vi "Rectangular Target - 2013Vr2.vi"(3 "Camera Settings":T4={"FPS"=30, "Compression"=30, "Image Size"=enum."320x240"}, 4 "Target Choice":i8(knob) scale=0.0..2.0, 5 "Camera IP Address":string="192.168.0.90", 6 "Camera Image":T2(plugin-control)) -> (0 "Center Target":bool, 1 "Processed Image":T2(plugin-control), 2 "Numeric Target Info":dbl[](array[numeric]))   [LabVIEW 2012]
doc: "This VI demonstrates how to do target processing on a laptop computer. It uses the same MJPG VI as the dashboard, sets a few of the important camera properties that impact processing, and carries out the same processing steps as the RT example also included in this project."
uses:
  <vilib>/Rock Robotics/WPI/Camera/WPI_CameraImageSize.ctl
  <vilib>/Rock Robotics/WPI/Camera/WPI_CameraWhite Balance Values.ctl
  <vilib>/vision/NI_Vision_Development_Module.lvlib
panel:
  in  "Camera Settings 2":T1={"Frate Rate"=30, "Compression"=30, "Size"=1} {"Size" items=["640x480", "320x240", "160x120"]; "Frate Rate" scale=1.0..30.0}
  out "fps":dbl format="%#.1g"
  in  "Camera Type":enum16{"206", "1011"}(ring)=enum."1011"
  in  "Image Source":enum32{"Live Camera", "File Images"}(tab)
  in  "Directory":path
  in  "File List":i32(listbox)
  out "Target Info":T5(array[cluster])
  in  "Area Size Limit %":dbl=0.5
  in  "Particle Count Limit":i32=10
  in  "Score Limits":T6={"Rect Coverage"=60.0, "X Edge Strength"=40.0, "Y Edge Strength"=60.0, "Center"=75.0, "Outer"=75.0}
  in  "Processing":enum32{"Color", "Monochrome"}(tab)
  out "Value":cluster{i32, i32}
  out "Saturation":cluster{i32, i32}
  in  "Value":i32=255
  in  "Saturation":i32=255
  in  "Hue":i32(knob)=65 scale=0.0..255.0
  in  "Margins":cluster{"Hue":i32, "Sat":i32, "Val":i32}={"Hue"=33, "Sat"=53, "Val"=9} {"Sat" scale=0.0..80.0; "Val" scale=0.0..80.0; "Hue" scale=0.0..80.0}
  out "Hue":cluster{i32, i32}
  in  "Range":cluster{"Lower value":sgl, "Upper value":sgl}={"Lower value"=150.0, "Upper value"=255.0} {"Lower value" scale=0.0..255.0; "Upper value" scale=0.0..255.0}
  in  "Color Plane":i32(ring)=6 items=["Red", "Green", "Blue", "Hue", "Saturation", "Luminance", "Value", "Intensity"]
  in  "Annotate":bool=TRUE
  out "Original Image":T2(plugin-control)
  # "Information:\nProcessing can be based on color or light intensity.\nParticles within the image are scored by rectangle coverage, aspect ratio, and\nedge strength/hollowness. A particle is considered a target if all scores\nare above the score limits you set. Particles can be annotated -- surrounded by\na rectangle and scores drawn to the left .\nTo control the number of particles being scored, use the count limit and the size\nlimit.\nBe sure to set the Camera IP before running. The distance calculation uses the\ncamera type to index the value of the lens view angle."
  # "Click in the image to choose  color for processing."
  # "Green scores are above the limit, orange are below. Inner/outer rect\nindicates all passed."
  # "Set before running."
  # "Lower/Upper"
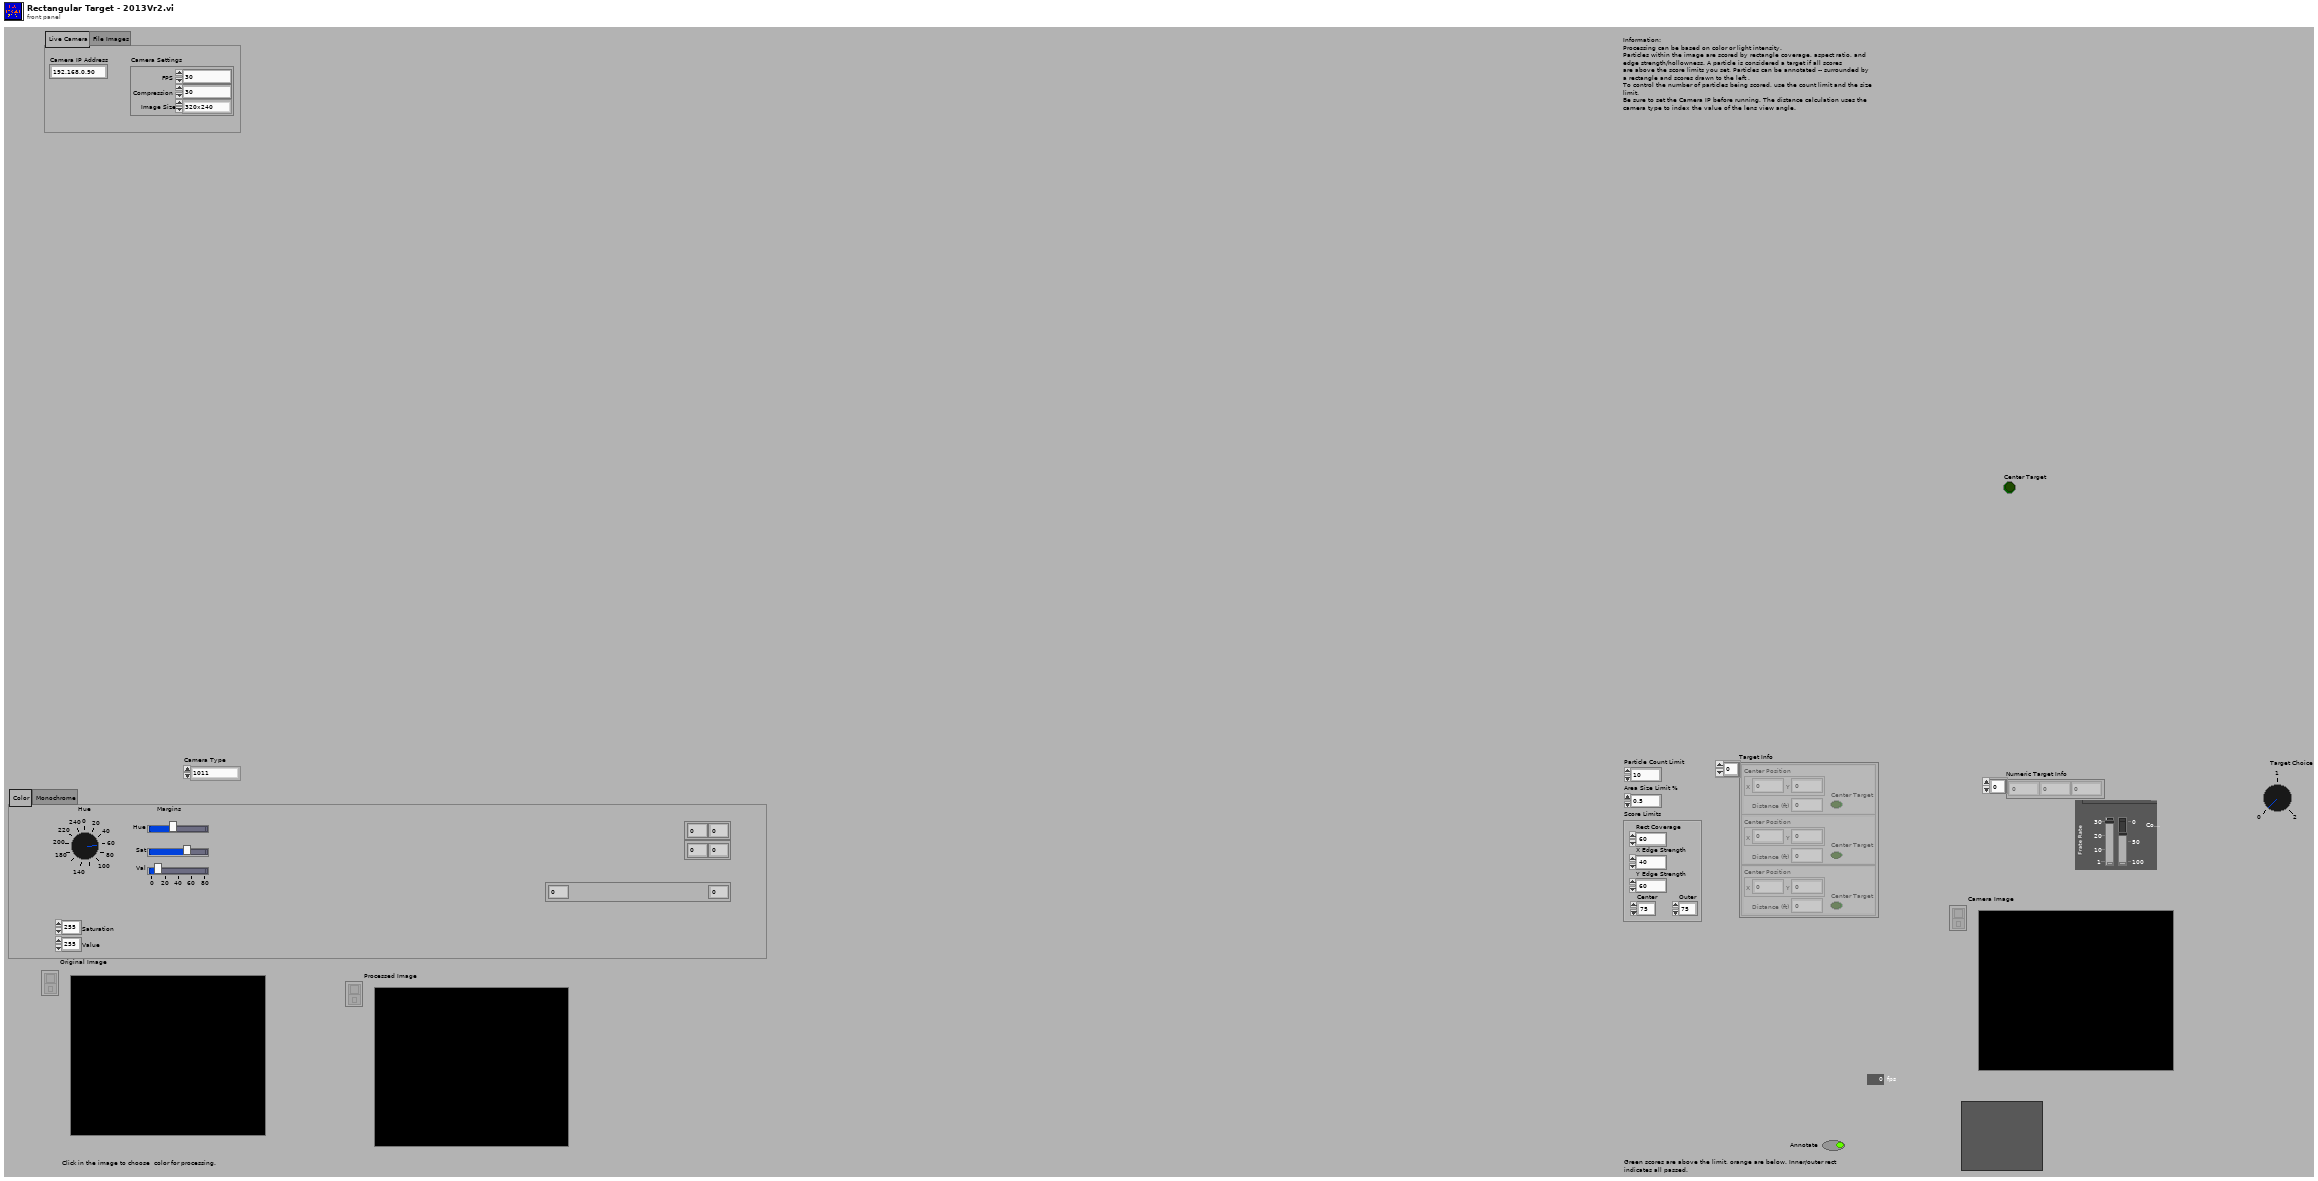
[diagram p1: front panel]
types:
  T1 = cluster{"Frate Rate":i32, "Compression":i32, "Size":u16}
  T2 = typedef "IMAQ Image.ctl" = refnum<image>
  T3 = typedef "WPI_CameraImageSize.ctl" = enum16{"640x480", "320x240", "160x120"}
  T4 = cluster{"FPS":i32, "Compression":i32, "Image Size":T3}
  T5 = cluster{"Center Position":cluster{"X":dbl, "Y":dbl}, "Distance (ft)":dbl, "Center Target":bool}[]
  T6 = cluster{"Rect Coverage":dbl, "X Edge Strength":dbl, "Y Edge Strength":dbl, "Center":dbl, "Outer":dbl}
  T7 = typedef "Image Type" = u32
  T8 = typedef "WPI_CameraWhite Balance Values.ctl" = enum16{"Auto", "Fixed indoor", "Fixed outdoor 1", "Fixed outdoor 2", "Fixed fluorescent 1", "Fixed fluorescent 2", "Hold current"}
  T9 = typedef "WPI_CameraDevRef.ctl" = cluster{"Camera Address":string, "CameraStatus":errorcluster, "Acquire Image Notifier":refnum<notifier>}
  T10 = cluster{"Position":cluster{"X":dbl, "Y":dbl}, "Distance (ft)":dbl, "Center Target":bool}[]
  T11 = cluster{cluster{"Left":dbl, "Top":dbl, "Right":dbl, "Bottom":dbl}, "Scores":dbl[], cluster{"Long":dbl, "Short":dbl}}[]
  T12 = cluster{"Target Center (-1 to 1)":cluster{"X":dbl, "Y":dbl}, "Distance (ft)":dbl, "Center Target":bool}
  T13 = cluster{"Target Center (-1 to 1)":cluster{"X":dbl, "Y":dbl}, "Distance (ft)":dbl, "Center Target":bool}[]
  T14 = cluster{"Left":dbl, "Top":dbl, "Right":dbl, "Bottom":dbl}
  T15 = cluster{"Position":cluster{"X":dbl, "Y":dbl}, "Distance (ft)":dbl, "Center Target":bool}
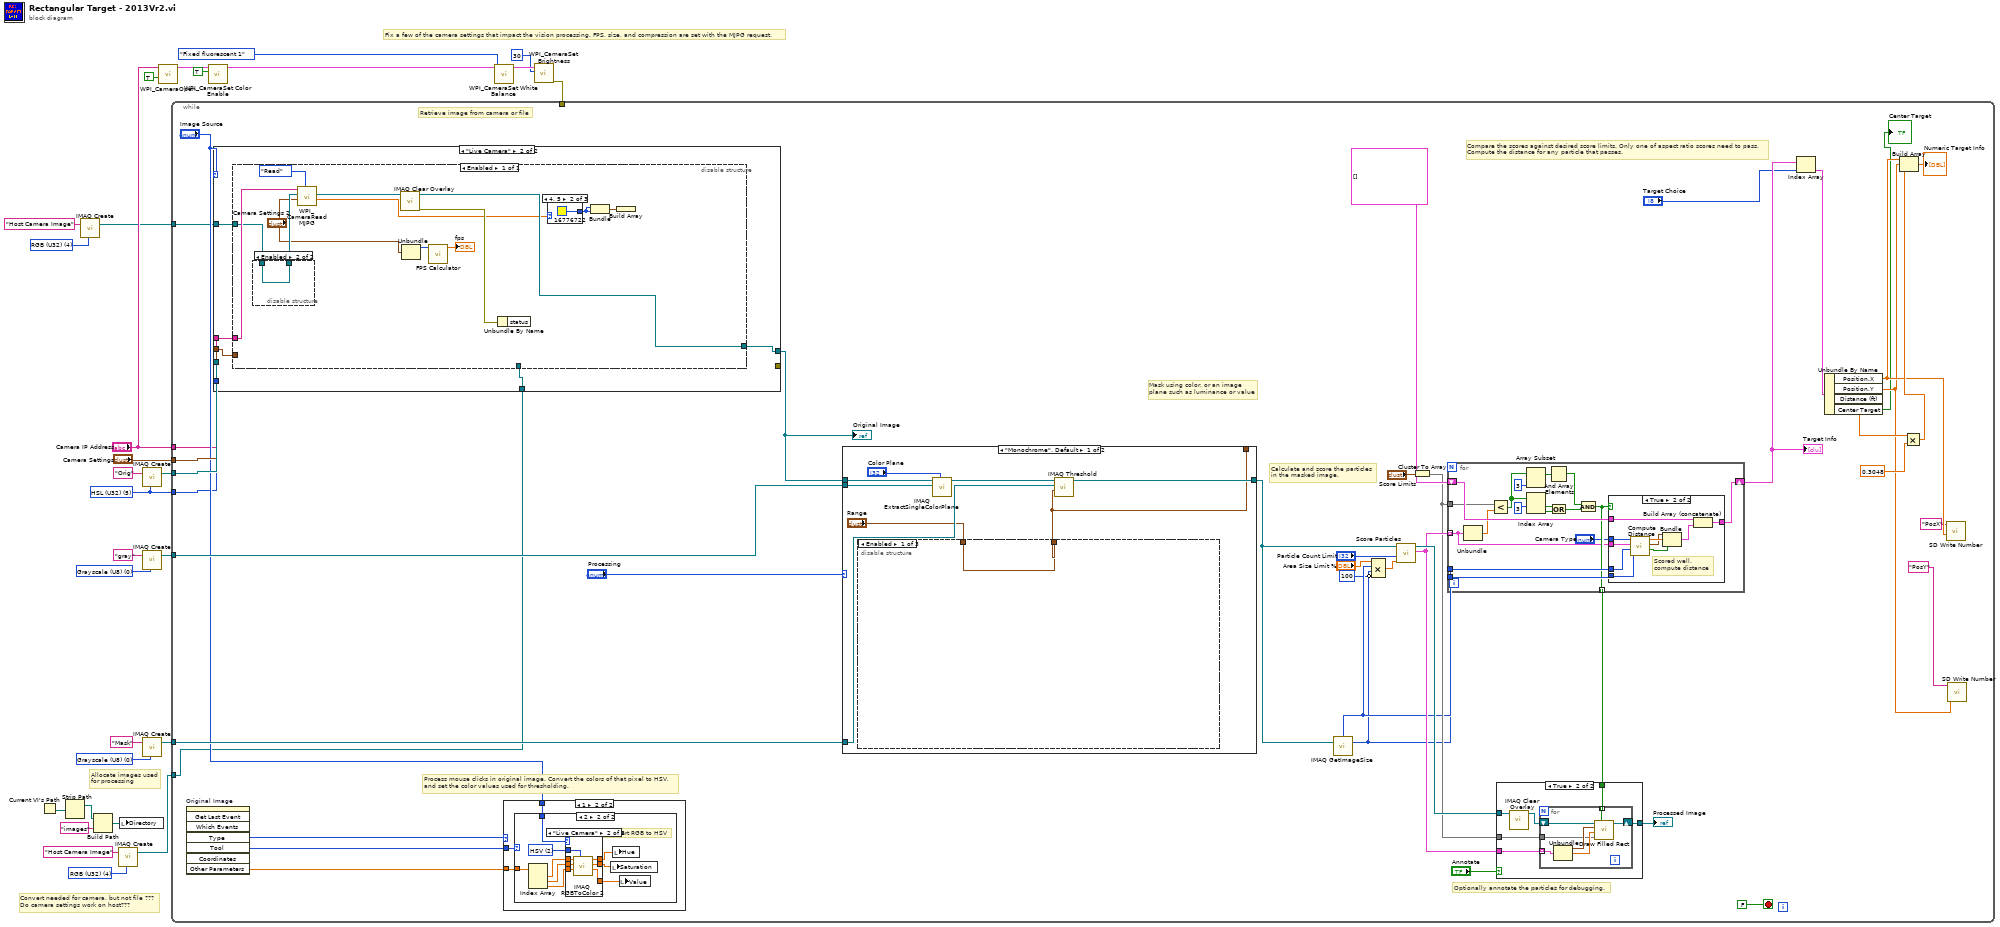
[diagram p0: block diagram]
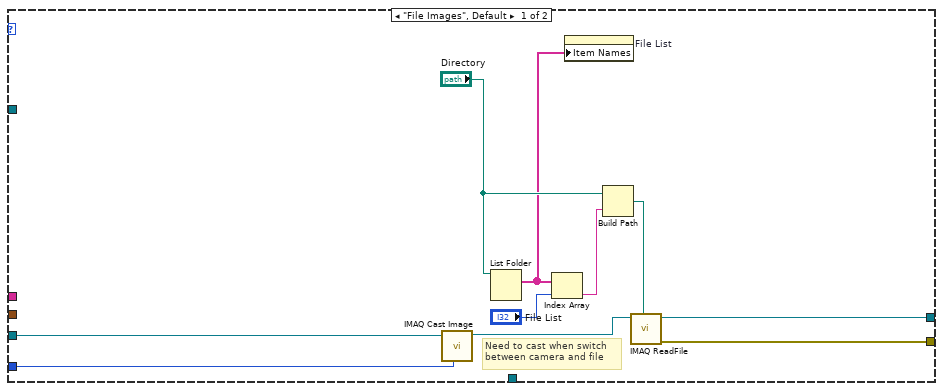
[diagram p2: hidden frame]
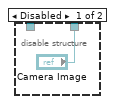
[diagram p3: hidden frame]
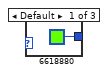
[diagram p4: hidden frame]
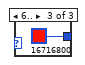
[diagram p5: hidden frame]
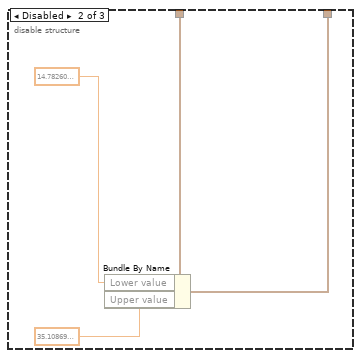
[diagram p7: hidden frame]
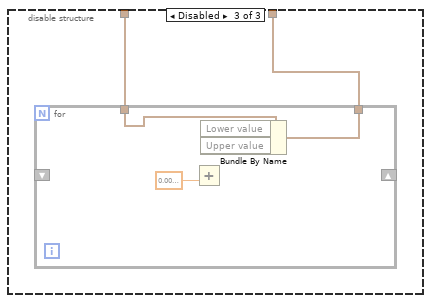
[diagram p8: hidden frame]
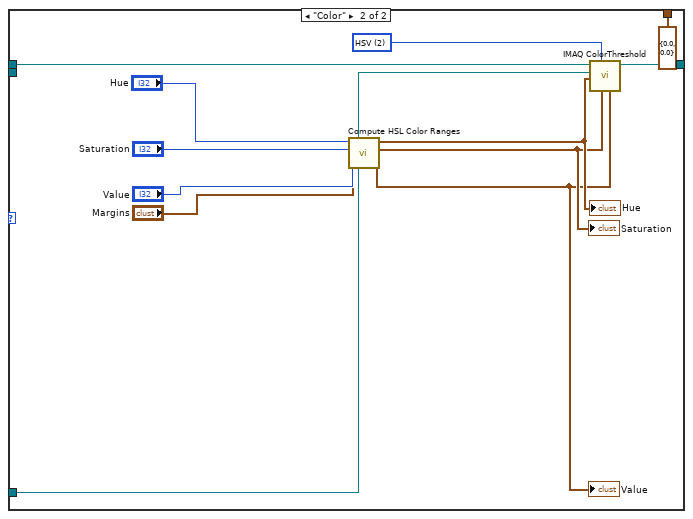
[diagram p9: hidden frame]
diagram:
  w3 = T7 4 items=["Grayscale (U8)", "Grayscale (I16)", "Grayscale (SGL)", "Complex (CSG)", "RGB (U32)", "HSL (U32)", "RGB (U64)"] ("Image Type")
  w7 = T7 4 items=["Grayscale (U8)", "Grayscale (I16)", "Grayscale (SGL)", "Complex (CSG)", "RGB (U32)", "HSL (U32)", "RGB (U64)"] ("Image Type")
  w23 = T7 0 items=["Grayscale (U8)", "Grayscale (I16)", "Grayscale (SGL)", "Complex (CSG)", "RGB (U32)", "HSL (U32)", "RGB (U64)", "Grayscale (U16)"] ("Image Type")
  w9 = T7 5 items=["Grayscale (U8)", "Grayscale (I16)", "Grayscale (SGL)", "Complex (CSG)", "RGB (U32)", "HSL (U32)", "RGB (U64)", "Grayscale (U16)"] ("Image Type")
  w29 = T7 0 items=["Grayscale (U8)", "Grayscale (I16)", "Grayscale (SGL)", "Complex (CSG)", "RGB (U32)", "HSL (U32)", "RGB (U64)", "Grayscale (U16)"] ("Image Type")
  # "Convert needed for camera, but not file ???\nDo camera settings work on host???"
  # "Allocate images used\nfor processing"
  # "Fix a few of the camera settings that impact the vision processing. FPS, size, and compression are set with the MJPG request."
  n1 = Current VI's Path() -> (path=w13:path)
  n2 = Strip Path(path=w13) -> (stripped path=w11:path)  [unwired: 1 out]
  n3 = call "IMAQ Create"("Image Name"="Host Camera Image", "Image Type"=w3) -> ("New Image"=w1:T2)  [unwired: 2 in, 2 out]
  n4 = Build Path(base path=w11, name or relative path="images") -> (appended path=w10:path)
  n5 = call "IMAQ Create"("Image Name"="Host Camera Image", "Image Type"=w7) -> ("New Image"=w5:T2)  [unwired: 2 in, 2 out]
  n6 = local write "Directory"(w10) -> ()
  n7 = call "IMAQ Create"("Image Name"="Orig", "Image Type"=w9) -> ("New Image"=w26:T2)  [unwired: 2 in, 2 out]
  n8 = call "IMAQ Create"("Image Name"="gray", "Image Type"=w29) -> ("New Image"=w25:T2)  [unwired: 2 in, 2 out]
  n9 = call "IMAQ Create"("Image Name"="Mask", "Image Type"=w23) -> ("New Image"=w22:T2)  [unwired: 2 in, 2 out]
  n10 = call <vilib>:"WPI_CameraOpen.vi"("Disallow Simulation"=TRUE, "Camera Address"="Camera IP Address") -> ("CameraDevRef"=w19:T9)  [unwired: 8 in, 1 out]
  n11 = call <vilib>:"WPI_CameraSet Color Enable.vi"("Color Enabled"=TRUE, "CameraDevRef"=w19) -> ("CameraDevRef Out"=w17:T9)  [unwired: 8 in, 1 out]
  n12 = call <vilib>:"WPI_CameraSet White Balance.vi"("White Balance"=WPI_CameraWhite_Balance_Values."Fixed fluorescent 1", "CameraDevRef"=w17) -> ("CameraDevRef Out"=w15:T9)  [unwired: 8 in, 1 out]
  n13 = call <vilib>:"WPI_CameraSet Brightness.vi"("Brightness"=30, "CameraDevRef"=w15) -> ("error out"=w21:errorcluster)  [unwired: 8 in, 1 out]
  n14 = while {
    tunnel: w26 -> [w65]
    tunnel: w25 -> [w71]
    tunnel: w22 -> [w52]
    tunnel: w21 -> [_]
    tunnel: "Camera Settings" -> [w55]
    tunnel: w9 -> [w50]
    tunnel: w5 -> [w33]
    tunnel: "Camera IP Address" -> [w32]
    tunnel: w1 -> [w30]
    stop <- FALSE stop-if-true
    # "Retrieve image from camera or file"
    # "Optionally annotate the particles for debugging."
    # "Compare the scores against desired score limits. Only one of aspect ratio scores need to pass.\nCompute the distance for any particle that passes."
    # "Process mouse clicks in original image. Convert the colors of that pixel to HSV,\nand set the color values used for thresholding."
    # "Calculate and score the particles\nin the masked image."
    # "Mask using color, or an image\nplane such as luminance or value"
    n15 = invoke on="Original Image" class="ImageControl" method="Get Last Event"() -> ("Type"=w66:i32, "Tool"=w67:i32, "Other Parameters"=w68:sgl[])  [unwired: 8 in, 5 out]
    n16 = case shown="\"Live Camera\"" "Image Source" {
      tunnel: w65 -> [w74 _]
      tunnel: [w81 w83] -> w64
      tunnel: w55 -> [_ w86]
      tunnel: [w80 _] -> _
      tunnel: w50 -> [w72 _]
      tunnel: w33 -> [_ w85]
      tunnel: w32 -> [_ w84]
      tunnel: w30 -> [_ w82]
      frame "File Images", Default {
        # "Need to cast when switch\nbetween camera and file"
        n17 = call "IMAQ Cast Image"("Image Type"=w72, "Image Src"=w74) -> ("Image Dst Out"=w73:T2)  [unwired: 8 in, 1 out]
        n18 = List Folder(path="Directory") -> (filenames=w75:string[])  [unwired: 3 in, 3 out]
        n19 = Index Array(array=w75, index="File List") -> (element=w78:string)
        n20 = property on="File List" class="LstBox (strict)"("Item Names"=w75) -> ()  [unwired: 2 in, 2 out]
        n21 = Build Path(base path="Directory", name or relative path=w78) -> (appended path=w77:path)
        n22 = call "IMAQ ReadFile"("File Path"=w77, "Image"=w73) -> ("error out"=w80:errorcluster, "Image Out"=w81:T2)  [unwired: 5 in, 3 out]
      }
      frame "Live Camera" {
        n23 = disable-structure shown="Enabled" {
          disable-tunnel: w86 -> [_]
          disable-tunnel: w85 -> [_]
          disable-tunnel: w84 -> [w98]
          disable-tunnel: [w95] -> w83
          disable-tunnel: w82 -> [w87]
          frame Enabled {
            n24 = disable-structure shown="Enabled" {
              disable-tunnel: ["Camera Image" w101] -> w99
              disable-tunnel: w87 -> [_ w101]
              frame Disabled {
              }
              frame Enabled {
              }
            }
            n25 = call <vilib>:"WPI_CameraRead MJPG.vi"("Operation"=enum16{"Read", "Reopen", "Close"}."Read", "Camera Settings"="Camera Settings 2", "Image"=w99, "address"=w98) -> ("Bandwidth (kbps)"=w88:dbl, "Image Out"=w96:T2)  [unwired: 5 in, 1 out]
            n26 = call "IMAQ Clear Overlay"("Image"=w96) -> ("error out"=w89:errorcluster, "Image Out"=w95:T2)  [unwired: 2 in, 7 out]
            n27 = Unbundle("Camera Settings 2") -> ("Frate Rate"=w93:i32)  [unwired: 2 out]
            n28 = call "FPS Calculator.vi"("Average Count"=w93) -> ("fps"=→"fps":dbl)  [unwired: 10 in]
            n29 = Unbundle By Name(w89) -> ()  [unwired: 1 out]
            n30 = case shown="4, 5" w88 {
              tunnel: [u32 6618880 ("Color Box") u32 16776722 ("Color Box") u32 16716800 ("Color Box")] -> w90
              frame Default {
              }
              frame 4, 5 {
              }
              frame 6.. {
              }
            }
            n31 = Bundle("Color Box"=w90, "Color Box"=w90) -> (w91:cluster{"Color Box":u32, "Color Box":u32})  [unwired: 1 out]
            n32 = Build Array(w91) -> ()  [unwired: 1 out]
          }
        }
      }
    }
    "Original Image" <- w64
    n33 = case shown="1" w66 {
      tunnel: w67 -> [_ w179]
      tunnel: w68 -> [_ w178]
      tunnel: "Image Source" -> [_ w177]
      frame 0, Default {
      }
      frame 1 {
        n34 = case shown="2" w179 {
          tunnel: w178 -> [_ w188]
          tunnel: w177 -> [_ w180]
          frame Default {
          }
          frame 2 {
            w187 = u16 2 items=["RGB", "HSL", "HSV", "HSI", "CIE L*a*b*", "CIE XYZ"] ("Color Mode")
            # "Convert RGB to HSV"
            n35 = Index Array(array=w188) -> (element #1=w186:sgl, element #2=w184:sgl, element #3=w182:sgl)  [unwired: 3 in]
            n36 = case shown="\"Live Camera\"" w180 {
              tunnel: w187 -> [_ w198]
              tunnel: w186 -> [w191 w197]
              tunnel: [w191 w196] -> w185
              tunnel: w184 -> [w190 w195]
              tunnel: [w190 w194] -> w183
              tunnel: w182 -> [w189 w193]
              tunnel: [w189 w192] -> w181
              frame "File Images", Default {
              }
              frame "Live Camera" {
                n37 = call "IMAQ RGBToColor 2"("Color Mode"=w198, "Blue value"=w193, "Green value"=w195, "Red value"=w197) -> ("Blue or Luma or Val or Inten or Z or b*value"=w192:dbl, "Green or Sat or Y or a* value"=w194:dbl, "Red or Hue or X or L* value"=w196:dbl)  [unwired: 4 in, 1 out]
              }
            }
            n38 = local write "Saturation"(w183) -> ()
            n39 = local write "Hue"(w185) -> ()
            n40 = local write "Value"(w181) -> ()
          }
        }
      }
    }
    n41 = case shown="\"Monochrome\", Default" "Processing" {
      tunnel: w64 -> [w126 w148]
      tunnel: w71 -> [w125 _]
      tunnel: [w123 w147] -> w58
      tunnel: w52 -> [w121 w139]
      tunnel: [w119 cluster{"Lower value":sgl, "Upper value":sgl} {"Lower value"=0.0, "Upper value"=0.0} ("Range")] -> _
      frame "Monochrome", Default {
        n42 = disable-structure shown="Enabled" {
          disable-tunnel: "Range" -> [w127 w129 w133]
          disable-tunnel: [w127 w128 w132] -> w119
          frame Enabled {
          }
          frame Disabled {
            n43 = Bundle By Name(cluster=w129, "Lower value"=sgl 14.7826, "Upper value"=sgl 35.1087) -> (w128:cluster{"Lower value":sgl, "Upper value":sgl})
          }
          frame Disabled {
            n44 = for {
              shift-right: _ -> [_]
              shift-left: _ -> [_]
              tunnel: w133 -> [w135]
              tunnel: [w134] -> w132
              n45 = Add(y=sgl 0.01) -> ()  [unwired: 1 in, 1 out]
              n46 = Bundle By Name(cluster=w135) -> (w134:cluster{"Lower value":sgl, "Upper value":sgl})  [unwired: 2 in]
            }
          }
        }
        n47 = call "IMAQ ExtractSingleColorPlane"("Color Plane"="Color Plane", "Image Dst"=w125, "Image Src"=w126) -> ("Image Dst Out"=w124:T2)  [unwired: 1 in, 7 out]
        n48 = call "IMAQ Threshold"("Range"=w119, "Image Dst"=w121, "Image Src"=w124) -> ("Image Dst Out"=w123:T2)  [unwired: 3 in, 5 out]
      }
      frame "Color" {
        w146 = u16 2 items=["RGB", "HSL", "HSV", "HSI"] ("Color Mode")
        n49 = call "Compute HSL Color Ranges.vi"("Margins"="Margins", "Luminance"="Value", "Saturation"="Saturation", "Hue"="Hue") -> ("Lum Range"=w140:cluster{i32, i32}, "Sat Range"=w141:cluster{i32, i32}, "Hue Range"=w145:cluster{i32, i32})  [unwired: 5 in]
        "Hue" <- w145
        "Saturation" <- w141
        "Value" <- w140
        n50 = call "IMAQ ColorThreshold"("Blue or Luma or Val or Inten Range"=w140, "Green or Sat Range"=w141, "Color Mode"=w146, "Red or Hue Range"=w145, "Image Dst"=w139, "Image Src"=w148) -> ("Image Dst Out"=w147:T2)  [unwired: 4 in, 1 out]
      }
    }
    n51 = call "IMAQ GetImageSize"("Image"=w58) -> ("Y Resolution"=w47:i32, "X Resolution"=w48:i32)  [unwired: 3 in, 1 out]
    n52 = Compound Arithmetic op=MULTIPLY("Area Size Limit %", w48, w47, invert 100 ("value")) -> (w46:dbl)
    n53 = call "Score Particles.vi"("Area Size Limit"=w46, "Particle Count Limit"="Particle Count Limit", "Image Refnum in"=w58) -> ("Scored Particle Info"=w60:T11, "Image Refnum out"=w63:T2)  [unwired: 7 in]
    n54 = Cluster To Array(cluster="Score Limits") -> (array=w54:dbl[])
    n55 = for {
      shift-right: [w164] -> w44
      shift-left: T10 [] -> [w165]
      tunnel: w48 -> [w163]
      tunnel: w60 -> [w149] mode=indexing
      tunnel: w54 -> [w161]
      tunnel: w47 -> [w160]
      tunnel: [w151] -> w53 mode=indexing
      n56 = Unbundle(w149) -> ("Scores"=w162:dbl[])  [unwired: 2 out]
      n57 = Less?(x=w161, y=w162) -> (x < y?=w157:bool[])
      n58 = Array Subset(array=w157, length=3) -> (w158:bool[])  [unwired: 1 in]
      n59 = Index Array(array=w157, index #1=3 ("length")) -> (element #1=w155:bool, element #2=w154:bool)  [unwired: 1 in]
      n60 = And Array Elements(Boolean array=w158) -> (logical AND=w152:bool)
      n61 = Or(x=w155, y=w154) -> (x .or. y?=w153:bool)
      n62 = And(x=w152, y=w153) -> (x .and. y?=w151:bool)
      n63 = case shown="True" w151 {
        tunnel: w165 -> [w166 w176]
        tunnel: [w166 w175] -> w164
        tunnel: w163 -> [_ w173]
        tunnel: "Camera Type" -> [_ w171]
        tunnel: w160 -> [_ w169]
        tunnel: w149 -> [_ w168]
        frame False {
          # "Didn't score well enough"
        }
        frame True {
          # "Scored well,\ncompute distance"
          n64 = call "Compute Distance.vi"("Y Image Resolution"=w169, "X Image Resolution"=w173, "Particle Scores"=w168, "Camera Type"=w171) -> ("Center Target"=w167:bool, "Target Center (-1 to 1)"=w170:cluster{"X":dbl, "Y":dbl}, "Distance (ft)"=w172:dbl)  [unwired: 5 in]
          n65 = Bundle("Target Center (-1 to 1)"=w170, "Distance (ft)"=w172, "Center Target"=w167) -> (w174:T12)  [unwired: 1 in]
          n66 = Build Array (concatenate)(w176, w174) -> (w175:T13)
        }
      }
    }
    "Target Info" <- w44
    n67 = case shown="True" "Annotate" {
      tunnel: w63 -> [w105 w111]
      tunnel: [w105 w110] -> w61
      tunnel: w60 -> [_ w108]
      tunnel: w54 -> [_ w107]
      tunnel: w53 -> [_ w106]
      frame False {
      }
      frame True {
        n68 = call "IMAQ Clear Overlay"("Image"=w111) -> ("Image Out"=w109:T2)  [unwired: 2 in, 8 out]
        n69 = for {
          shift-right: [w117] -> w110
          shift-left: w109 -> [w118]
          tunnel: w108 -> [w114] mode=indexing
          tunnel: w107 -> [w113]
          tunnel: w106 -> [w112] mode=indexing
          n70 = Unbundle(w114) -> (w115:T14, "Scores"=w116:dbl[])  [unwired: 1 out]
          n71 = call "Draw Filled Rect.vi"("Limit Passed"=w112, "Limits"=w113, "Scores"=w116, "Bounding Box"=w115, "image in"=w118) -> ("image out"=w117:T2)  [unwired: 6 in]
        }
      }
    }
    "Processed Image" <- w61
    n72 = Index Array(array=w44, index="Target Choice") -> (element=w42:T15)
    n73 = Unbundle By Name(w42) -> ("Position.X"=w37:dbl, "Position.Y"=w36:dbl, "Distance (ft)"=w41:dbl, "Center Target"=→"Center Target":bool)
    n74 = Multiply(x=w41, y=0.3048) -> (x*y=w39:dbl)
    n75 = Build Array(w37, w36, w39) -> (→"Numeric Target Info":dbl[])
    n76 = call <vilib>:"SD Write Number.vi"("Numeric"=w37, "Name"="PosX") -> ()  [unwired: 8 in, 2 out]
    n77 = call <vilib>:"SD Write Number.vi"("Numeric"=w36, "Name"="PosY") -> ()  [unwired: 8 in, 2 out]
  }
